vi "Global_ACT_Data Out.vi"() -> ()   [LabVIEW 2020, in "Tube Wheel_ACT.lvlib"]
uses:
  Tube Wheel_ACT.lvlib
  Type Defs/ENUM_Tube Wheel CMD Positions.ctl
  Shared Code/TypeDefs/ENUM_Tube Wheel Positions.ctl
panel:
  out "At Target Position":bool
  in  "Current Position":T1
  in  "Target Position":T2
  in  "ACT_TubeWheel_Motor Value":dbl
  in  "ACT_TubeWheel_CycleTime(S)":dbl
  in  "ACT_TubeWheel_Count":i32
  # "The Names of the Data items in the Global Variable MUST describe who the Single Writer is\nFor Actuator Globals the the naming convention is\n   \nACT_Lib Name_Data Name\n\nExamples:\nACT_Drive_X axis\nACT_Hopper_AgitatorSpeed"
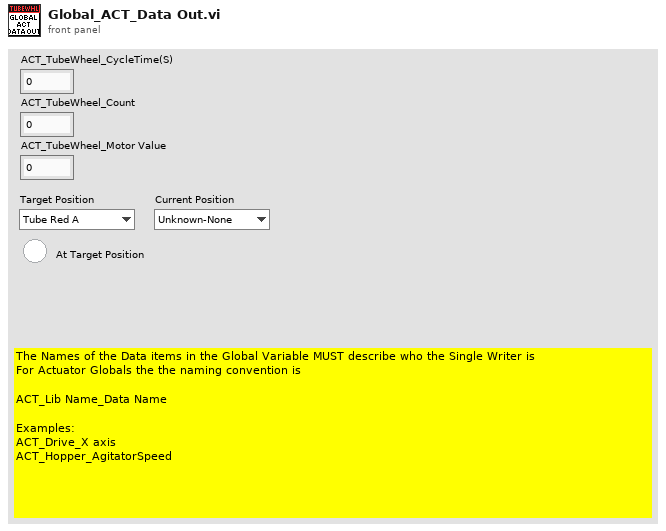
[diagram p1: front panel]
types:
  T1 = typedef "ENUM_Tube Wheel Positions.ctl" = enum16{"Unknown-None", "Tube Red A", "Tube Black B", "Tube Red C", "Tube Black D", "Tube Red E", "Tube Black F", "Load A-B", "Load B-C", "Load C-D", "Load D-E", "Load E-F", "Load F-A"}
  T2 = typedef "ENUM_Tube Wheel CMD Positions.ctl" = enum16{"Tube Red A", "Tube Black B", "Tube Red C", "Tube Black D", "Tube Red E", "Tube Black F"}
diagram:
